vi "append_log.vi"(1 "Prepend Timestamp (T)":bool=TRUE, 2 "New Log String":string) -> (0 "Log":string)   [LabVIEW 2011]
uses:
  globals.vi
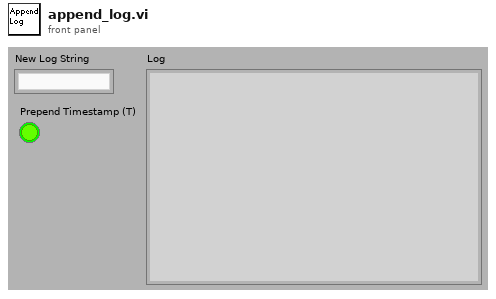
[diagram p1: front panel]
types:
  T1 = enum16{"open", "replace", "create", "open or create", "replace or create", "replace or create with confirmation"}
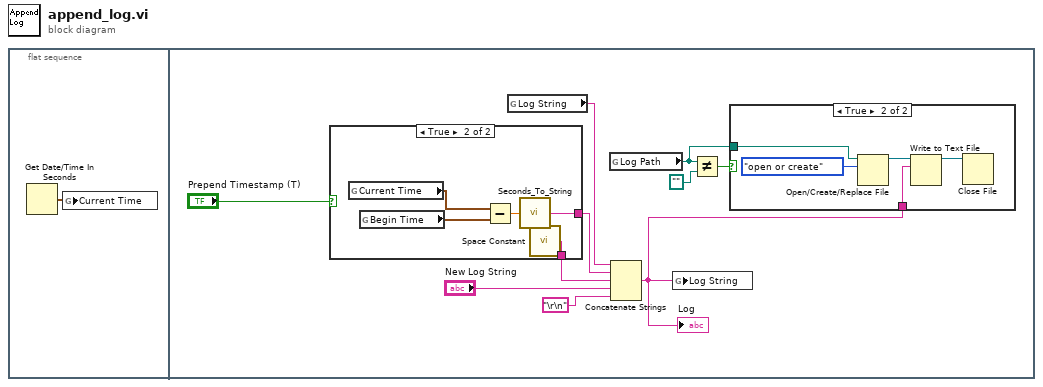
[diagram p0: block diagram]
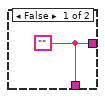
[diagram p3: hidden frame]
diagram:
  n1 = flat-sequence {
    frame #0 {
      n2 = Get Date/Time In Seconds() -> (seconds since 1Jan1904=w1:timestamp)
      n3 = global write "globals.vi" "Current Time"(w1) -> ()
    }
    frame #1 {
      n4 = case shown="True" "Prepend Timestamp (T)" {
        tunnel: [w17 w22] -> w10
        tunnel: [w17 w18] -> w7
        frame False {
          w17 = ""
        }
        frame True {
          n5 = global read "globals.vi" "Current Time"() -> (w19:timestamp)
          n6 = global read "globals.vi" "Begin Time"() -> (w20:timestamp)
          n7 = Subtract(x=w19, y=w20) -> (x-y=w21:dbl)
          n8 = call "Seconds_To_String.vi"("Seconds"=w21) -> ("Output String"=w22:string)
          n9 = call <vilib>:"Space Constant.vi"() -> ("String"=w18:string)
        }
      }
      n10 = global read "globals.vi" "Log String"() -> (w3:string)
      n11 = global read "globals.vi" "Log Path"() -> (w4:path)
      n12 = Concatenate Strings(w3, w10, w7, "New Log String", "\r\n") -> (w2:string)
      "Log" <- w2
      n13 = global write "globals.vi" "Log String"(w2) -> ()
      n14 = Not Equal?(x=w4, y=path "") -> (x != y?=w5:bool)
      n15 = case shown="True" w5 {
        tunnel: w4 -> [_ w16]
        tunnel: w2 -> [_ w14]
        frame False {
        }
        frame True {
          n16 = Open/Create/Replace File(file path (use dialog)=w16, operation (0:open)=T1."open or create") -> (refnum out=w13:refnum<file>)  [unwired: 4 in, 2 out]
          n17 = Write to Text File(file (use dialog)=w13, text=w14) -> (refnum out=w12:refnum<file>)  [unwired: 2 in, 2 out]
          n18 = Close File(refnum=w12) -> ()  [unwired: 1 in, 2 out]
        }
      }
    }
  }
